vi "wyborSciezki.vi"(6 "error in (no error)":errorcluster, 9 "Path Control":path) -> (0 "error out":errorcluster, 3 "Path Indicator":path)   [LabVIEW 2017]
panel:
  in  "OK Button":bool
  # "Wybór ścieżki"
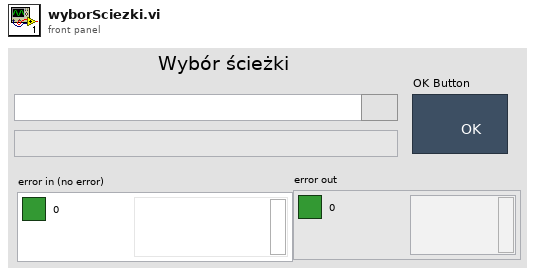
[diagram p1: front panel]
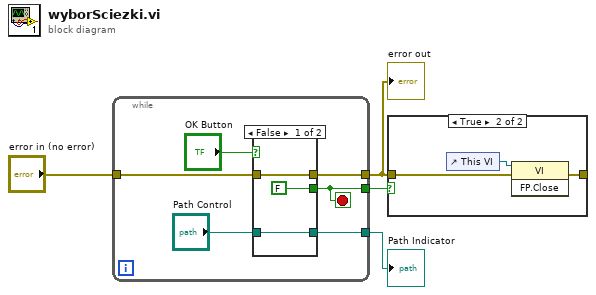
[diagram p0: block diagram]
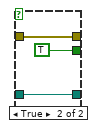
[diagram p3: hidden frame]
diagram:
  n1 = while {
    tunnel: [w8] -> w4
    tunnel: [w7] -> w1
    tunnel: "error in (no error)" -> [w6]
    tunnel: [w5] -> w2
    stop <- w5 stop-if-true
    n2 = case shown="False" "OK Button" {
      tunnel: "Path Control" -> [w11 w15]
      tunnel: w6 -> [w13 w16]
      tunnel: [w13 w16] -> w7
      tunnel: [w11 w15] -> w8
      tunnel: [FALSE TRUE] -> w5
      frame False {
      }
      frame True {
      }
    }
  }
  "Path Indicator" <- w4
  "error out" <- w1
  n3 = case shown="True" w2 {
    tunnel: w1 -> [_ w19]
    tunnel: [_ w18] -> _
    frame False {
    }
    frame True {
      n4 = control-ref of="This VI"() -> (w17:refnum<vi>)
      n5 = invoke class="VI" method="FP.Close"(reference=w17, error in=w19) -> (error out=w18:errorcluster)  [unwired: 1 in, 2 out]
    }
  }
